vi "Receive Dashboard Packet.vi"(7 "connection ID":refnum<k16>) -> ()   [LabVIEW 2014]
uses:
  Common Code/Dashboard Control Data.ctl
  Common Code/Roller Control.ctl
  Common Code/Elevator DB Control.ctl
  Robot Global Data.vi
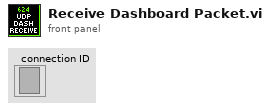
[diagram p1: front panel]
types:
  T1 = typedef "Dashboard Control Data.ctl" = cluster{"Cam Exposure":dbl, "Go to angle":dbl, "Steer PID Gains":cluster{"proportional gain (Kc)":dbl, "integral time (Ti, min)":dbl, "derivative time (Td, min)":dbl}, "Steer PID output Range":cluster{"output high":dbl, "output low":dbl}, "Pressure m \nValue":dbl, "Pressure b \nValue":dbl, "Strafe Timer\nWait":dbl, "Roller Command Cluster ":T2, "Elevator":T3, "Strafe Correct min X":dbl}
  T2 = typedef "Roller Control.ctl" = cluster{"Left Roller Speed":dbl, "Right Roller Speed":dbl, "Left Roller Speed Back":dbl, "Right Roller Speed Back":dbl, "Roller Align Decide Limit":u32}
  T3 = typedef "Elevator DB Control.ctl" = cluster{"Presets":cluster{"Hold Tote":dbl, "Hold Trashcan":dbl, "Pickup 2 w/ Tote":dbl, "Pickup 2 w/ Trashcan":dbl, "Pickup 3 w/ Tote":dbl, "Pickup 3 w/ Trashcan":dbl, "Lift Plate Deploy":dbl, "Bottom":dbl, "Lift Plate Deploy for 2":dbl, "Lift Plate Deploy for 3":dbl}, "PID Output Range":cluster{"output high":dbl, "output low":dbl}, "PID gains":cluster{"proportional gain (Kc)":dbl, "integral time (Ti, min)":dbl, "derivative time (Td, min)":dbl}, "LP Close Angle":i32, "LP Open Angle":i32, "Height Tolerance":dbl, "L Encoder Constant":dbl, "R Encoder Constant":dbl}
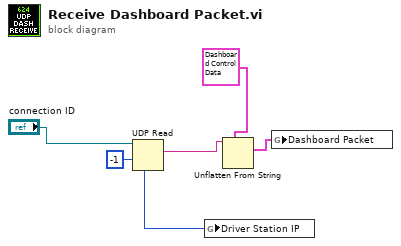
[diagram p0: block diagram]
diagram:
  n1 = UDP Read(connection ID="connection ID", timeout ms (25000)=-1) -> (data out=w6:string, 6:w3:u32)  [unwired: 2 in, 3 out]
  n2 = global write "Robot Global Data.vi" "Driver Station IP"(w3) -> ()
  n3 = Unflatten From String(type=T1 {"Cam Exposure"=0.0, "Go to angle"=0.0, "Steer PID Gains"={"proportional gain (Kc)"=1.0, "integral time (Ti, min)"=0.01, "derivative time (Td, min)"=0.0}, "Steer PID output Range"={"output high"=1.0, "output low"=-1.0}, "Pressure m \nValue"=0.0, "Pressure b \nValue"=0.0, "Strafe Timer\nWait"=0.0, "Roller Command Cluster "={"Left Roller Speed"=0.0, "Right Roller Speed"=0.0, "Left Roller Speed Back"=0.0, "Right Roller Speed Back"=0.0, "Roller Align Decide Limit"=1000}, "Elevator"={"Presets"={"Hold Tote"=0.0, "Hold Trashcan"=0.0, "Pickup 2 w/ Tote"=0.0, "Pickup 2 w/ Trashcan"=0.0, "Pickup 3 w/ Tote"=0.0, "Pickup 3 w/ Trashcan"=0.0, "Lift Plate Deploy"=0.0, "Bottom"=0.0, "Lift Plate Deploy for 2"=0.0, "Lift Plate Deploy for 3"=0.0}, "PID Output Range"={"output high"=100.0, "output low"=-100.0}, "PID gains"={"proportional gain (Kc)"=1.0, "integral time (Ti, min)"=0.01, "derivative time (Td, min)"=0.0}, "LP Close Angle"=0, "LP Open Angle"=0, "Height Tolerance"=0.0, "L Encoder Constant"=0.0, "R Encoder Constant"=0.0}, "Strafe Correct min X"=0.0} ("DB Control Data"), binary string=w6) -> (value=w4:T1)  [unwired: 3 in, 2 out]
  n4 = global write "Robot Global Data.vi" "Dashboard Packet"(w4) -> ()
